vi "通信原理实验任务 1_2何德轩.vi"(1 "bitstream":i32[](array[numeric])) -> (0 "output":i32)   [LabVIEW 2018]
panel:
  out "boolean array":bool[](array[boolean])
  # "将二进制数组转化为一个十进制数值"
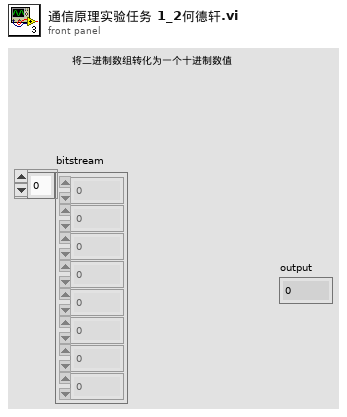
[diagram p1: front panel]
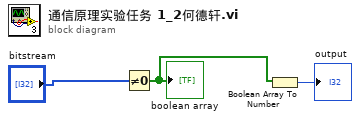
[diagram p0: block diagram]
diagram:
  n1 = Not Equal To 0?(x="bitstream") -> (x != 0?=w2:bool[])
  "boolean array" <- w2
  n2 = Boolean Array To Number(Boolean array=w2) -> (number=→"output":u32)
